vi "Right Gripper Missed.vi"(6 "Gripper Opening":sgl, 9 "Object Size":sgl) -> ()   [LabVIEW 2013]
uses:
  ROS/Code/SubVIs/BaxterSide.ctl
panel:
  in  "continue":bool
  in  "Gripper":bool
  # "Gripper Missed Object"
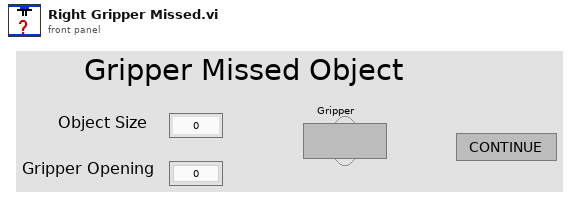
[diagram p1: front panel]
types:
  T1 = typedef "BaxterSide.ctl" = enum16{"left", "right"}
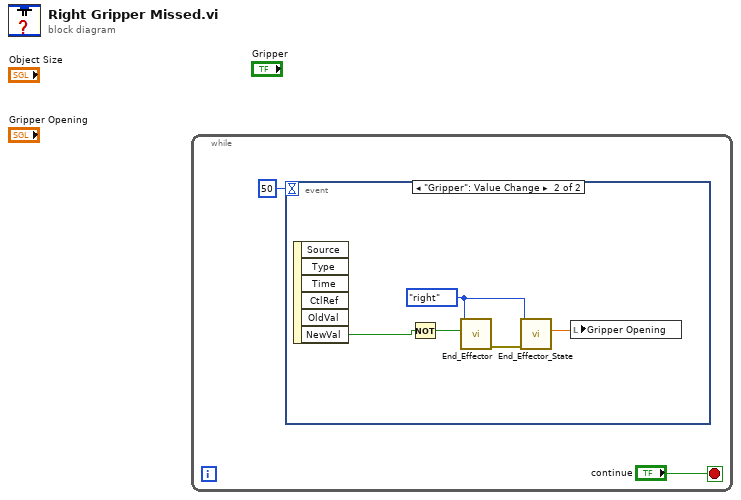
[diagram p0: block diagram]
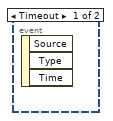
[diagram p2: hidden frame]
diagram:
  n1 = while {
    stop <- "continue" stop-if-true
    n2 = event shown="[1] \"Gripper\": Value Change" {
      selector: _ -> [_ _]
      dyn-events: _ -> [_ _]
      timeout: 50 -> [_ _]
      event Timeout {
        n3 = event-data() -> ()  [unwired: 1 in, 3 out]
      }
      event "Gripper": Value Change {
        w5 = BaxterSide."right" ("Side")
        n4 = event-data() -> ("NewVal"=w4:bool)  [unwired: 1 in, 5 out]
        n5 = Not(x=w4) -> (.not. x?=w6:bool)
        n6 = call "End_Effector.vi"("Close"=w6, "Side"=w5) -> ("error out"=w7:errorcluster)  [unwired: 6 in]
        n7 = call "End_Effector_State.vi"("error in"=w7, "Side"=w5) -> ("position"=w3:sgl)  [unwired: 3 in, 3 out]
        n8 = local write "Gripper Opening"(w3) -> ()
      }
    }
  }
